vi "Auto-Refresh Tester.vi"() -> ()   [LabVIEW 2014, in "SimSyA.lvlib"]
uses:
  SimSyA.lvlib
  DriverMasterSync/build/DriverMasterSync.lvlibp/APIs/Data Queue/Acquisition Data 1 Sample Cluster.ctl
  DriverMasterSync/build/DriverMasterSync.lvlibp/APIs/Data Queue/Control Data Cluster.ctl
  SimSyAClass/SimSyA.lvclass
  DriverMasterSync/build/DriverMasterSync.lvlibp/APIs/Data Queue/WINFAS 2 Data Queue.lvlib
panel:
  out "Control Data":T1
  out "1 Sample":T2
  in  "stop":bool
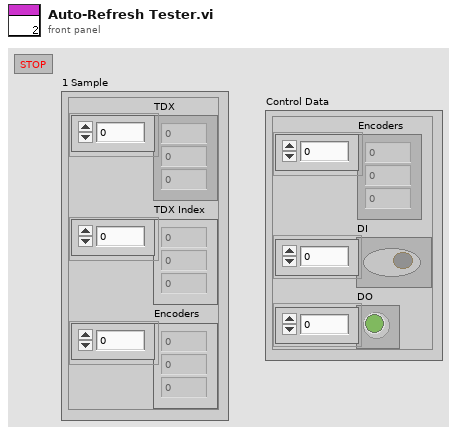
[diagram p1: front panel]
types:
  T1 = typedef "DriverMasterSync.lvlibp/WINFAS 2 Data Queue.lvlib/Control Data Cluster.ctl" = cluster{"Encoders":i32[], "DI":bool[], "DO":bool[]}
  T2 = typedef "DriverMasterSync.lvlibp/WINFAS 2 Data Queue.lvlib/Acquisition Data 1 Sample Cluster.ctl" = cluster{"TDX":sgl[], "TDX Index":u32[], "Encoders":i32[]}
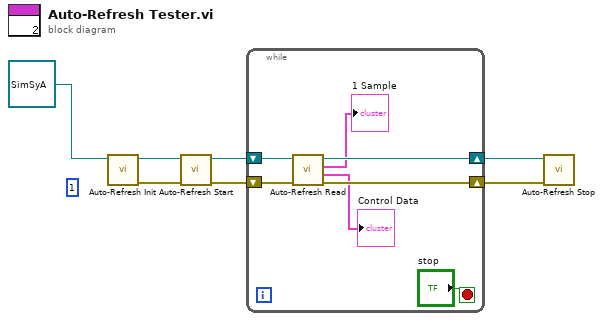
[diagram p0: block diagram]
diagram:
  (unwired) u64 1 ("Channel Mask")
  n1 = call-dynamic "Auto-Refresh Init.vi"("SimSyA in"=refnum<class "SimSyA.lvclass"> refnum) -> ("error out"=w3:errorcluster, "SimSyA out"=w7:refnum<class "SimSyA.lvclass">)  [unwired: 9 in]
  n2 = call-dynamic "Auto-Refresh Start.vi"("error in (no error)"=w3, "SimSyA in"=w7) -> ("error out"=w2:errorcluster, "SimSyA out"=w6:refnum<class "SimSyA.lvclass">)  [unwired: 8 in]
  n3 = while {
    shift-right: [w13] -> w4
    shift-left: w6 -> [w14]
    shift-right: [w11] -> w1
    shift-left: w2 -> [w12]
    stop <- "stop" stop-if-true
    n4 = call-dynamic "Auto-Refresh Read.vi"("error in (no error)"=w12, "SimSyA in"=w14) -> ("error out"=w11:errorcluster, "Control Data"=→"Control Data":T1, "1 Sample"=→"1 Sample":T2, "SimSyA out"=w13:refnum<class "SimSyA.lvclass">)  [unwired: 6 in]
  }
  n5 = call-dynamic "Auto-Refresh Stop.vi"("error in (no error)"=w1, "SimSyA in"=w4) -> ()  [unwired: 8 in, 2 out]
